vi "VI Main 1.2.vi"() -> ()   [LabVIEW 2014]
uses:
  <vilib>/Analysis/NI_AALPro.lvlib
panel:
  in  "Array":bool[](array[boolean])
  out "None linear Intervals":dbl[](array[numeric])
  out "Measuring! 2":bool
  in  "Residue Threshold":dbl=2.0 format="%.3g"
  in  "Gain":dbl=3.31
  in  "Offset":dbl=-0.032 step=0.01 format="%_3f"
  in  "K1":dbl=-2.995 format="%#_13g"
  in  "K0":dbl=0.9054 format="%#_13g"
  in  "samples/channel":i32=10
  in  "Rate (Hz)":dbl=100.0
  in  "DAQ channels":tag="Dev2/ai23"
  in  "RH/T Sensor VSS (V)":dbl=2.0 format="%.3g"
  out "residue":dbl
  in  "COM:":bool
  in  "clear graph at start":bool=TRUE
  in  "clear graph":bool
  out "Elapsed Time":dbl=5.100291728973389 format="%<%H:%M:%S>t"
  out "Measuring!":bool
  out "Current Interval":i32=2
  out "Benchmark (s)":dbl=1.077 format="%.2g"
  out "Start time":timestamp=timestamp(3634319869.0891385 s since 1904-01-01)
  in  "STOP acq":bool
  in  "# of Intervals":i32=20 min=2 step=1
  in  "Interval (s)":dbl=3.0 min=1.0 step=1.0
  in  "Quick Acq":bool
  in  "Multi Acq":bool
  in  "Reset":bool
  in  "Single Acq":bool
  in  "stop":bool
  out "intercept":dbl=5.632151768673284e-07 format="%_4g"
  out "Waveform Chart":dbl(graph)
  out "Res. (ohm)":dbl=1498.8953969009954 format="%#.5g"
  out "XY Graph":cluster{dbl[], "Best Linear Fit":dbl[]}[](graph)=[{[0.0, 0.05050000175833702, 0.10100000351667404, 0.15150000154972076, 0.20200000703334808, 0.2524999976158142, 0.30300000309944153, 0.35350000858306885, 0.40400001406669617, 0.4544999897480011, 0.5049999952316284, 0.5554999709129333, 0.6060000061988831, 0.656499981880188, 0.7070000171661377, 0.7574999928474426, 0.8080000281333923, 0.8585000038146973, 0.9089999794960022, 0.9595000147819519, 1.0099999904632568, 1.0605000257492065, 1.1109999418258667, 1.1614999771118164, 1.2120000123977661, 1.2625000476837158, 1.312999963760376, 1.3634999990463257, 1.4140000343322754, 1.4644999504089355, 1.5149999856948853, 1.565500020980835, 1.6160000562667847, 1.6664999723434448, 1.7170000076293945, 1.7675000429153442, 1.8179999589920044, 1.868499994277954, 1.9190000295639038, 1.969499945640564, 2.0199999809265137, 2.070499897003174, 2.121000051498413, 2.1714999675750732, 2.2219998836517334, 2.2725000381469727, 2.322999954223633, 2.373500108718872, 2.4240000247955322, 2.4744999408721924, 2.5255000591278076, 2.5759999752044678, 2.626499891281128, 2.677000045776367, 2.7274999618530273, 2.7780001163482666, 2.8285000324249268, 2.878999948501587, 2.929500102996826, 2.9800000190734863, 3.0304999351501465, 3.0810000896453857, 3.131500005722046, 3.181999921798706, 3.2325000762939453, 3.2829999923706055, 3.3334999084472656, 3.384000062942505, 3.434499979019165, 3.484999895095825, 3.5355000495910645, 3.5859999656677246, 3.6364998817443848, 3.687000036239624, 3.737499952316284, 3.7880001068115234, 3.8385000228881836, 3.8889999389648438, 3.939500093460083, 3.990000009536743, 4.040500164031982, 4.091000080108643, 4.141499996185303, 4.191999912261963, 4.242499828338623, 4.293000221252441, 4.343500137329102, 4.394000053405762, 4.444499969482422, 4.494999885559082, 4.545499801635742, 4.5960001945495605, 4.646500110626221, 4.697000026702881, 4.747499942779541, 4.797999858856201, 4.848499774932861, 4.89900016784668, 4.94950008392334, 5.0], "Best Linear Fit"=[2.9321361694201187e-07, 3.4316144592594355e-05, 6.788442260585725e-05, 0.00010163152910536155, 0.0001353666593786329, 0.0001692490477580577, 0.00020289691747166216, 0.0002365230757277459, 0.0002702110796235502, 0.0003039317671209574, 0.0003375497763045132, 0.00037135041202418506, 0.00040501810144633055, 0.000438651826698333, 0.0004723611054942012, 0.0005059913382865489, 0.0005397166823968291, 0.0005734616424888372, 0.0006071235402487218, 0.0006408520275726914, 0.000674474285915494, 0.0007079437491483986, 0.0007418016903102398, 0.0007753406534902751, 0.0008092316566035151, 0.0008428616565652192, 0.0008766247192397714, 0.0009101884788833559, 0.0009441068395972252, 0.000977773917838931, 0.0010113242315128446, 0.00104525254573673, 0.0010786742204800248, 0.0011119291884824634, 0.0011458882363513112, 0.0011792887235060334, 0.0012128128437325358, 0.001246674102731049, 0.0012809749459847808, 0.0013138956855982542, 0.0013484194641932845, 0.0013821402098983526, 0.001415521022863686, 0.0014488088199868798, 0.0014823464443907142, 0.0015171199338510633, 0.0015507071511819959, 0.0015843959990888834, 0.0016174258198589087, 0.001652282546274364, 0.001685628667473793, 0.001718429964967072, 0.0017526380252093077, 0.0017857326893135905, 0.0018194534350186586, 0.001854273141361773, 0.0018880483694374561, 0.0019207267323508859, 0.0019549881108105183, 0.001989204902201891, 0.0020224947948008776, 0.002056337194517255, 0.0020900650415569544, 0.0021233297884464264, 0.0021574627608060837, 0.0021917179692536592, 0.0022237151861190796, 0.002258580643683672, 0.0022912463173270226, 0.0023252873215824366, 0.0023596647661179304, 0.0023923530243337154, 0.0024269770365208387, 0.0024603772908449173, 0.002494191052392125, 0.0025280059780925512, 0.0025607654824852943, 0.0025952423457056284, 0.0026286595966666937, 0.0026625576429069042, 0.002696041017770767, 0.002730145351961255, 0.0027635691221803427, 0.0027978394646197557, 0.00283193145878613, 0.0028640953823924065, 0.002898684237152338, 0.0029313690029084682, 0.002965638181194663, 0.0029995907098054886, 0.0030326275154948235, 0.0030669174157083035, 0.003100987756624818, 0.003135110717266798, 0.0031680287793278694, 0.0032008818816393614, 0.0032355813309550285, 0.003269442357122898, 0.0033022440038621426, 0.0033363213296979666]}, {[0.0, 0.05050000175833702, 0.10100000351667404, 0.15150000154972076, 0.20200000703334808, 0.2524999976158142, 0.30300000309944153, 0.35350000858306885, 0.40400001406669617, 0.4544999897480011, 0.5049999952316284, 0.5554999709129333, 0.6060000061988831, 0.656499981880188, 0.7070000171661377, 0.7574999928474426, 0.8080000281333923, 0.8585000038146973, 0.9089999794960022, 0.9595000147819519, 1.0099999904632568, 1.0605000257492065, 1.1109999418258667, 1.1614999771118164, 1.2120000123977661, 1.2625000476837158, 1.312999963760376, 1.3634999990463257, 1.4140000343322754, 1.4644999504089355, 1.5149999856948853, 1.565500020980835, 1.6160000562667847, 1.6664999723434448, 1.7170000076293945, 1.7675000429153442, 1.8179999589920044, 1.868499994277954, 1.9190000295639038, 1.969499945640564, 2.0199999809265137, 2.070499897003174, 2.121000051498413, 2.1714999675750732, 2.2219998836517334, 2.2725000381469727, 2.322999954223633, 2.373500108718872, 2.4240000247955322, 2.4744999408721924, 2.5255000591278076, 2.5759999752044678, 2.626499891281128, 2.677000045776367, 2.7274999618530273, 2.7780001163482666, 2.8285000324249268, 2.878999948501587, 2.929500102996826, 2.9800000190734863, 3.0304999351501465, 3.0810000896453857, 3.131500005722046, 3.181999921798706, 3.2325000762939453, 3.2829999923706055, 3.3334999084472656, 3.384000062942505, 3.434499979019165, 3.484999895095825, 3.5355000495910645, 3.5859999656677246, 3.6364998817443848, 3.687000036239624, 3.737499952316284, 3.7880001068115234, 3.8385000228881836, 3.8889999389648438, 3.939500093460083, 3.990000009536743, 4.040500164031982, 4.091000080108643, 4.141499996185303, 4.191999912261963, 4.242499828338623, 4.293000221252441, 4.343500137329102, 4.394000053405762, 4.444499969482422, 4.494999885559082, 4.545499801635742, 4.5960001945495605, 4.646500110626221, 4.697000026702881, 4.747499942779541, 4.797999858856201, 4.848499774932861, 4.89900016784668, 4.94950008392334, 5.0], "Best Linear Fit"=[5.632151768673284e-07, 3.425469348999516e-05, 6.794617180312299e-05, 0.00010163764763089373, 0.00013532912842937865, 0.0001690205992864352, 0.00020271208008492013, 0.00023640356088340506, 0.00027009504168188996, 0.0003037865025975182, 0.0003374779833960031, 0.00037116944431163135, 0.0004048609449929729, 0.00043855240590860115, 0.0004722439065899428, 0.000505935367505571, 0.0005396268681869126, 0.0005733183291025409, 0.0006070097900181691, 0.0006407012906995107, 0.0006743927516151388, 0.0007080842522964805, 0.0007417756734463953, 0.0007754671741277369, 0.0008091586748090786, 0.0008428501754904202, 0.000876541596640335, 0.0009102330973216766, 0.0009439245980030183, 0.000977616019152933, 0.0010113075198342747, 0.0010449990205156163, 0.001078690521196958, 0.0011123819423468728, 0.0011460734430282144, 0.001179764943709556, 0.0012134563648594707, 0.0012471478655408123, 0.001280839366222154, 0.0013145307873720688, 0.0013482222880534104, 0.0013819137092033252, 0.0014156052894160936, 0.0014492967105660085, 0.0014829881317159233, 0.0015166797119286917, 0.0015503711330786066, 0.001584062713291375, 0.0016177541344412898, 0.0016514455555912046, 0.0016854706906080038, 0.0017191621117579187, 0.0017528535329078335, 0.001786545113120602, 0.0018202365342705167, 0.0018539281144832852, 0.0018876195356332, 0.0019213109567831148, 0.001955002536995883, 0.001988693958145798, 0.0020223853792957127, 0.0020560769595084813, 0.002089768380658396, 0.002123459801808311, 0.002157151382021079, 0.0021908428031709943, 0.002224534224320909, 0.0022582258045336775, 0.002291917225683592, 0.002325608646833507, 0.0023593002270462754, 0.00239299164819619, 0.002426683069346105, 0.0024603746495588733, 0.0024940660707087883, 0.0025277576509215565, 0.0025614490720714716, 0.002595140493221386, 0.002628832073434155, 0.0026625234945840694, 0.002696215074796838, 0.0027299064959467527, 0.0027635979170966677, 0.0027972893382465823, 0.0028309807593964974, 0.002864672498672119, 0.0028983639198220342, 0.002932055340971949, 0.002965746762121864, 0.0029994381832717785, 0.0030331296044216935, 0.0030668213436973154, 0.0031005127648472304, 0.003134204185997145, 0.0031678956071470596, 0.0032015870282969747, 0.0032352784494468893, 0.0032689701887225115, 0.003302661609872426, 0.003336353031022341]}]
  in  "Sense range":i32(slide)
  in  "Stop (V)":dbl=5.0 format="%.4f"
  in  "Source compliance (A)":dbl=0.01 format="%.4f"
  in  "Direction":i32(slide)
  in  "Ranging":i32(slide)
  in  "Start (V)":dbl step=1.0 format="%.4p"
  in  "# of points to acquire":i32=50 min=1 max=2500 step=1
  in  "Speed":i32(slide)=2
  out "status":i32 format="%.0x"
  in  "resource GPIB":string="GPIB0::24::INSTR"
  in  "resource RS232":string="ASRL4::INSTR"
  out "Qrun":bool
  out "Mrun":bool
  out "Srun":bool
  # ">"
  # "RH%/T Sensor"
  # "Ethanol Sensor"
  # "by L.Andrzejewski\nlandrzej@uottawa.ca"
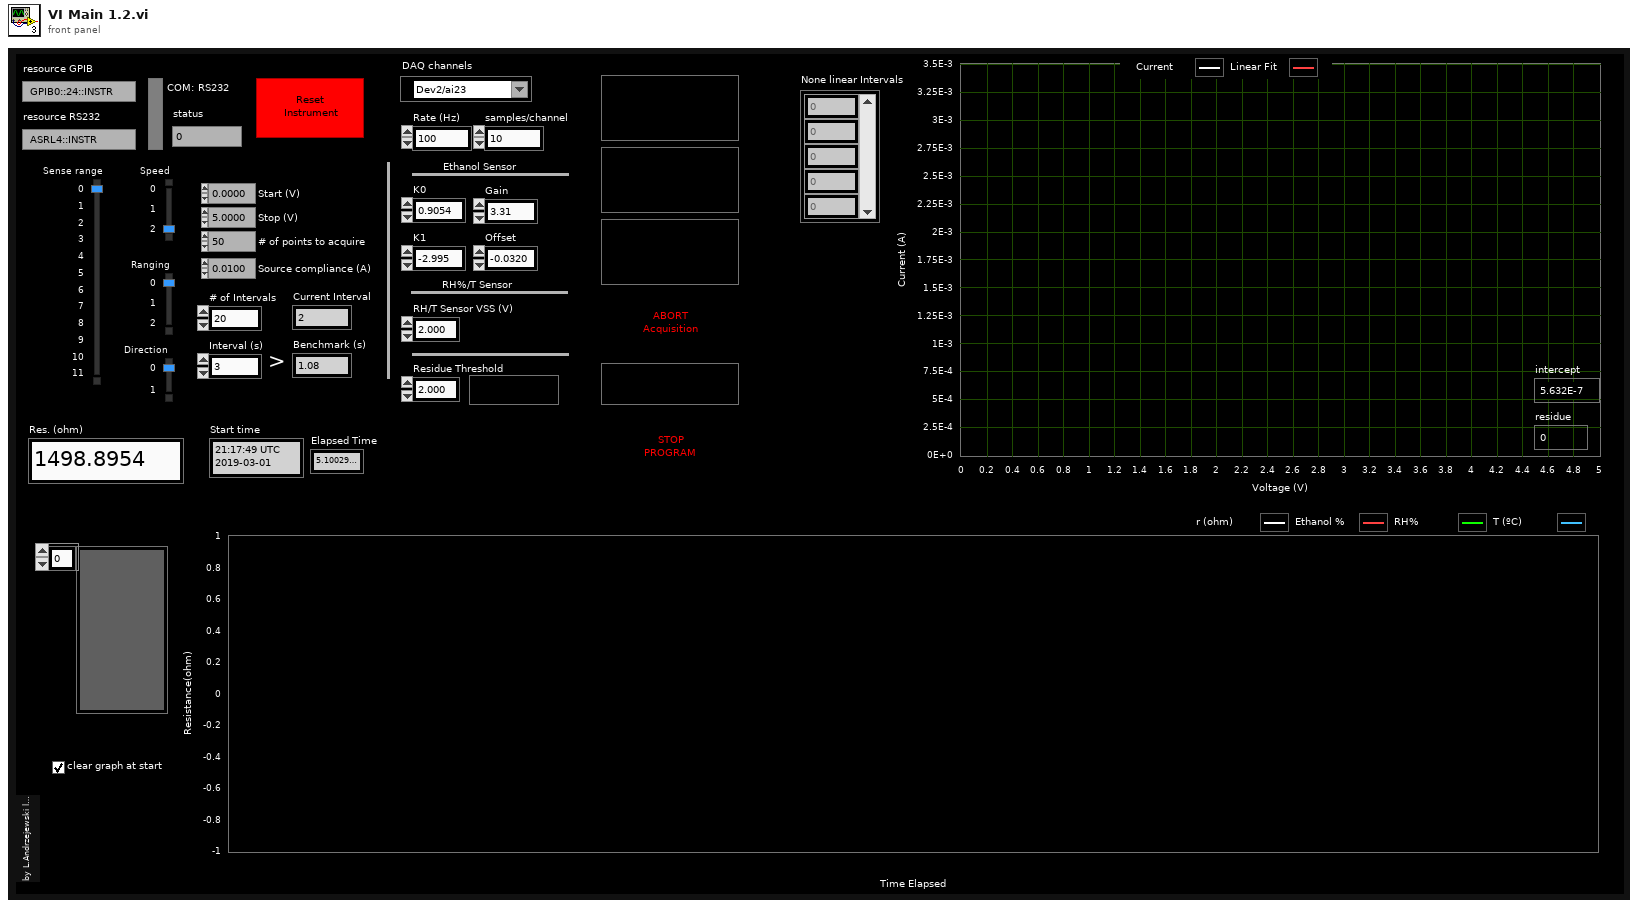
[diagram p1: front panel]
types:
  T1 = enum8{"Enabled", "Disabled", "Disabled and Grayed Out"}
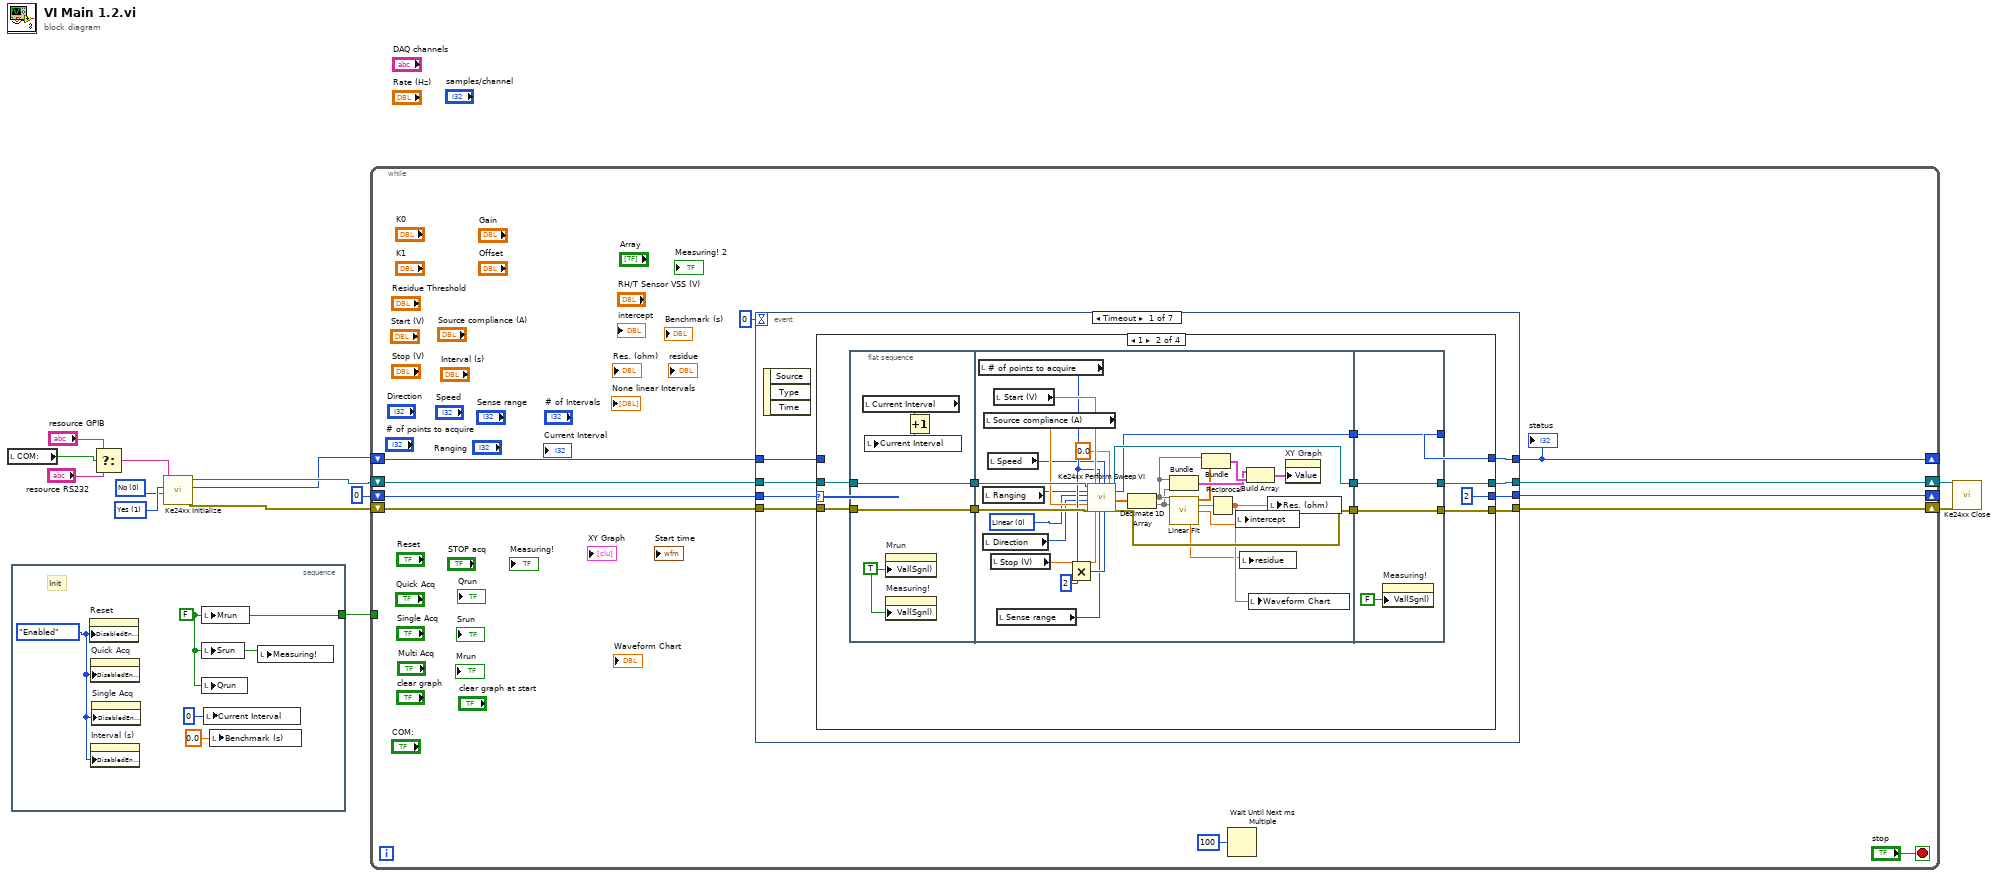
[diagram p0: block diagram]
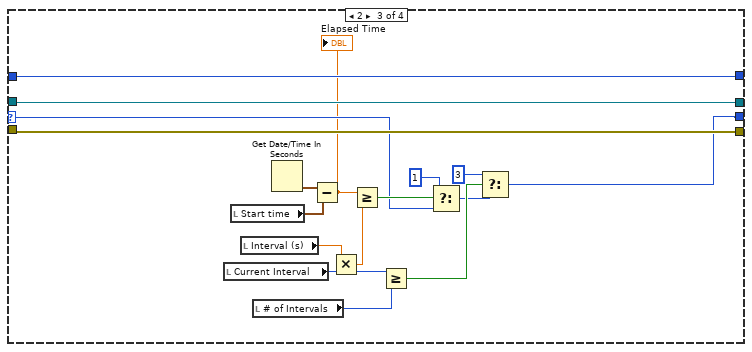
[diagram p3: hidden frame]
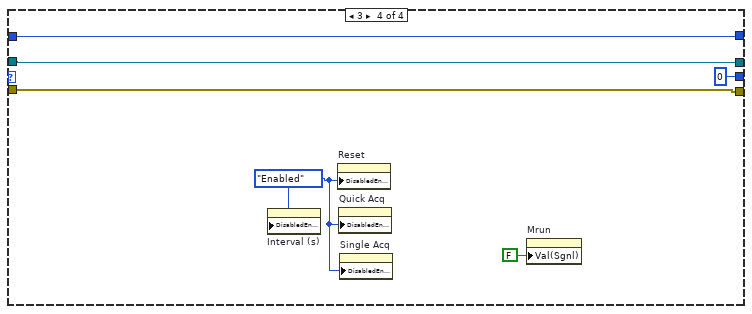
[diagram p4: hidden frame]
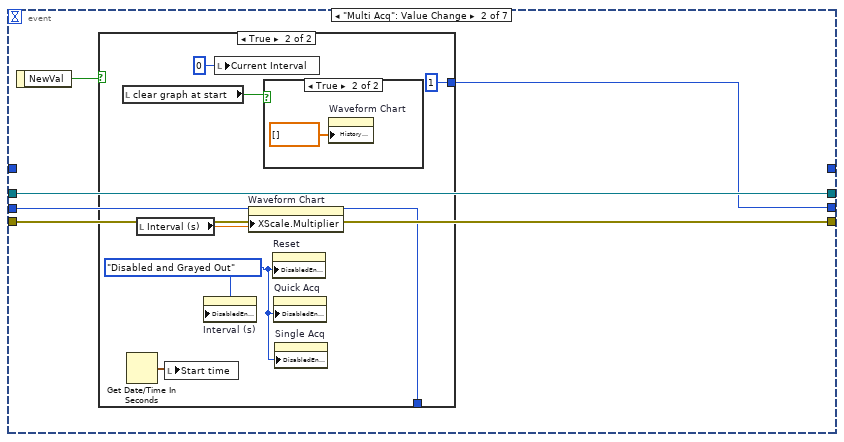
[diagram p5: hidden frame]
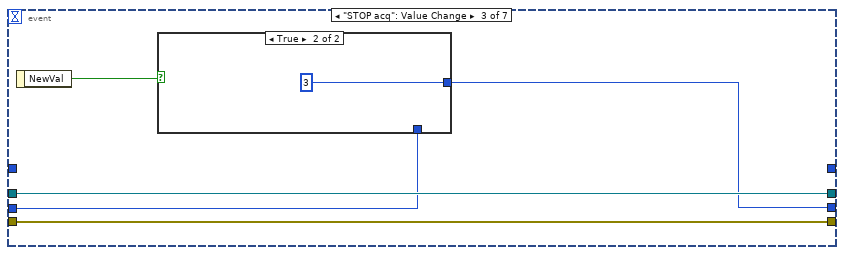
[diagram p8: hidden frame]
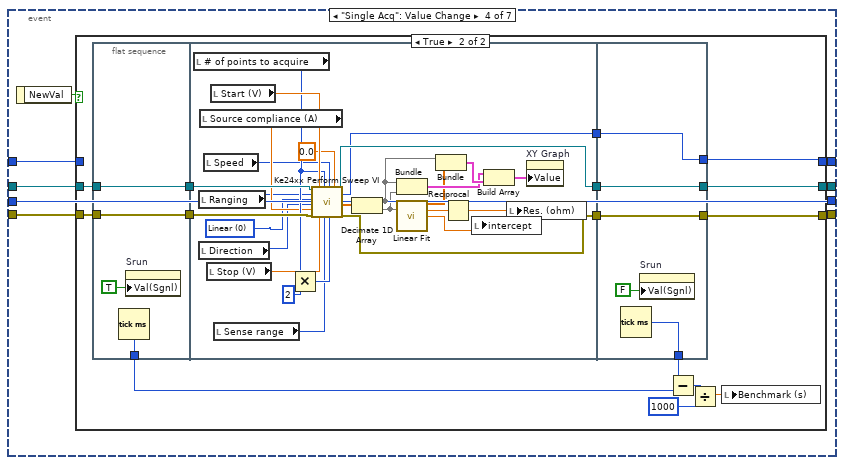
[diagram p10: hidden frame]
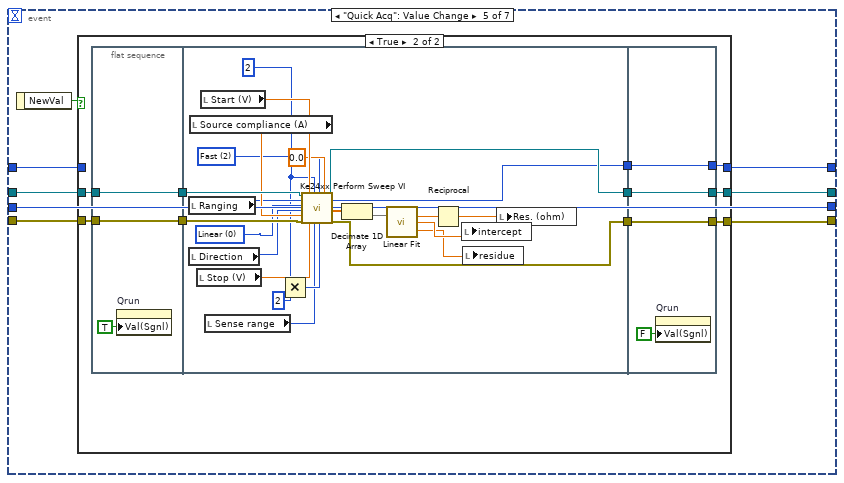
[diagram p12: hidden frame]
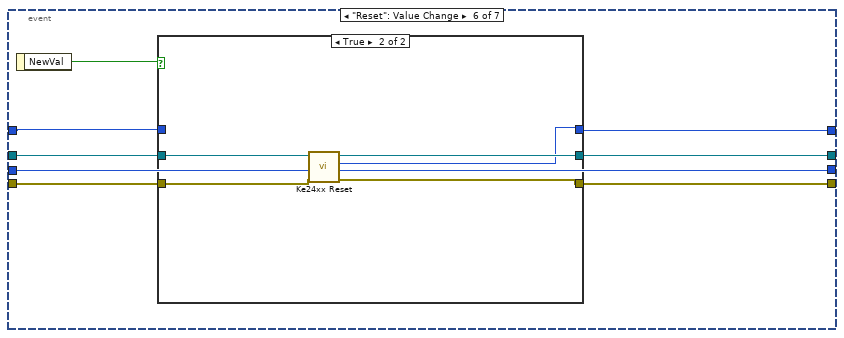
[diagram p14: hidden frame]
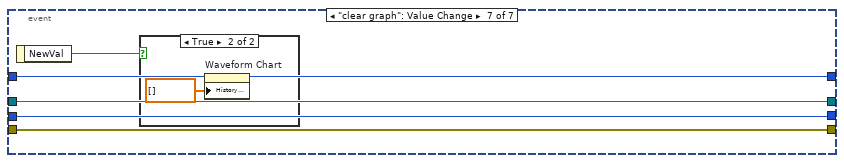
[diagram p16: hidden frame]
diagram:
  w13 = u16 1 items=["Yes"=1, "No"=0] ("id query")
  w5 = u16 0 items=["Yes"=1, "No"=0] ("reset device")
  n1 = local read "COM:"() -> (w4:bool)
  n2 = stacked-sequence {
    tunnel: [w15] -> w7
    frame #0 {
      w14 = T1."Enabled" ("Disabled")
      w15 = FALSE ("Mrun")
      # "Init"
      n3 = property on="Reset" class="Bool"("DisabledEnum"=w14) -> ()  [unwired: 2 in, 2 out]
      n4 = property on="Quick Acq" class="Bool"("DisabledEnum"=w14) -> ()  [unwired: 2 in, 2 out]
      n5 = property on="Interval (s)" class="DigNum (strict)"("DisabledEnum"=w14) -> ()  [unwired: 2 in, 2 out]
      n6 = property on="Single Acq" class="Bool"("DisabledEnum"=w14) -> ()  [unwired: 2 in, 2 out]
      n7 = local write "Mrun"(w15) -> ()
      n8 = local write "Srun"(w15) -> ()
      n9 = local write "Qrun"(w15) -> ()
      n10 = local write "Current Interval"(0 ("Current Interval")) -> ()
      n11 = local write "Benchmark (s)"(0.0 ("Benchmark (s)")) -> ()
      n12 = local write "Measuring!"(w15) -> ()
    }
  }
  n13 = Select(t="resource GPIB", s=w4, f="resource RS232") -> (s? t:f=w1:string)
  n14 = call <instrlib>:"Ke24xx Initialize.vi"("reset device"=w5, "id query"=w13, "resource name"=w1) -> ("error out"=w8:errorcluster, "status"=w9:i32, "instrument handle out"=w10:refnum<visa-resource-name>)  [unwired: 6 in]
  n15 = while {
    shift-right: [w23] -> w12
    shift-left: w10 -> [w25]
    shift-right: [w22] -> w11
    shift-left: w8 -> [w24]
    shift-right: [w20] -> _
    shift-left: w9 -> [w21]
    tunnel: w7 -> [_]
    shift-right: [w18] -> _
    shift-left: 0 -> [w19]
    stop <- "stop" stop-if-true
    n16 = event shown="[0] Timeout" {
      selector: _ -> [_ _ _ _ _ _ _]
      dyn-events: _ -> [_ _ _ _ _ _ _]
      timeout: 0 -> [_ _ _ _ _ _ _]
      tunnel: [w32 w115 w128 w135 w197 w249 w264] -> w23
      tunnel: w25 -> [w35 w115 w128 w138 w200 w250 w264]
      tunnel: [w31 w114 w127 w136 w198 w248 w262] -> w22
      tunnel: w24 -> [w34 w114 w127 w137 w199 w247 w262]
      tunnel: w21 -> [w33 _ _ w134 w196 w252 w265]
      tunnel: [w29 _ _ w133 w195 w251 w265] -> w20
      tunnel: w19 -> [w36 w112 w125 w132 w194 w246 w263]
      tunnel: [w30 w113 w126 w132 w194 w246 w263] -> w18
      event Timeout {
        n17 = event-data() -> ()  [unwired: 1 in, 3 out]
        n18 = case shown="1" w36 {
          selector: w36 -> [w37 _ w94 _]
          tunnel: w35 -> [w39 w49 w103 w109]
          tunnel: w34 -> [w38 w48 w104 w107]
          tunnel: w33 -> [w40 _ w105 w110]
          tunnel: [w39 w47 w103 w109] -> w32
          tunnel: [w38 w46 w104 w107] -> w31
          tunnel: [w37 2 w91 0 ("t")] -> w30
          tunnel: [w40 w44 w105 w110] -> w29
          frame 0, Default {
          }
          frame 1 {
            n19 = flat-sequence {
              tunnel: w48 -> [w55]
              tunnel: w49 -> [w56]
              tunnel: [w56] -> w51
              tunnel: [w55] -> w50
              tunnel: w51 -> [w77]
              tunnel: w50 -> [w76]
              tunnel: [w75] -> w43
              tunnel: [w74] -> w42
              tunnel: [w59] -> w41
              tunnel: [w86] -> w44
              tunnel: [w87] -> w47
              tunnel: [w88] -> w46
              tunnel: w43 -> [w88]
              tunnel: w42 -> [w87]
              tunnel: w41 -> [w86]
              frame #0 {
                w52 = TRUE ("Value (Signaling)")
                n20 = local read "Current Interval"() -> (w53:i32)
                n21 = property on="Mrun" class="Bool (strict)"("Val(Sgnl)"=w52) -> ()  [unwired: 2 in, 2 out]
                n22 = property on="Measuring!" class="Bool (strict)"("Val(Sgnl)"=w52) -> ()  [unwired: 2 in, 2 out]
                n23 = Increment(x=w53) -> (x+1=w54:i32)
                n24 = local write "Current Interval"(w54) -> ()
              }
              frame #1 {
                w61 = 0 items=["Linear", "Logarithmic"] ("spacing")
                n25 = local read "# of points to acquire"() -> (w68:i32)
                n26 = local read "Ranging"() -> (w63:i32)
                n27 = local read "Direction"() -> (w62:i32)
                n28 = local read "Source compliance (A)"() -> (w65:dbl)
                n29 = local read "Speed"() -> (w64:i32)
                n30 = local read "Stop (V)"() -> (w70:dbl)
                n31 = local read "Start (V)"() -> (w71:dbl)
                n32 = local read "Sense range"() -> (w66:i32)
                n33 = Multiply(x=w68, y=2) -> (x*y=w67:i32)
                n34 = call <instrlib>:"Ke24xx Perform Sweep VI.vi"("instrument handle"=w77, "ranging"=w63, "spacing"=w61, "direction"=w62, "source compliance"=w65, "error in (no error)"=w76, "start"=w71, "stop"=w70, "number of points"=w68, "sense range"=w66, "speed"=w64, "size of reading"=w67, "source protection"=0.0) -> ("instrument handle out"=w74:refnum<visa-resource-name>, "status"=w59:i32, "out"=w78:dbl[], "error out"=w75:errorcluster)  [unwired: 3 in]
                n35 = Decimate 1D Array(w78) -> (w82:dbl[], w79:dbl[])
                n36 = Bundle(w82, w79) -> (w83:cluster{dbl[], dbl[]})  [unwired: 1 in]
                n37 = call <vilib>:"Linear Fit.vi"("Y"=w79, "X"=w82) -> ("Best Linear Fit"=w81:dbl[], "slope"=w80:dbl, "intercept"=w73:dbl, "residue"=w57:dbl)  [unwired: 9 in, 1 out]
                n38 = Bundle(w82, "Best Linear Fit"=w81) -> (w84:cluster{dbl[], "Best Linear Fit":dbl[]})  [unwired: 1 in]
                n39 = Reciprocal(x=w80) -> (1/x=w58:dbl)
                n40 = local write "intercept"(w73) -> ()
                n41 = local write "residue"(w57) -> ()
                n42 = Build Array(w83, w84) -> (w72:cluster{dbl[], "Best Linear Fit":dbl[]}[])
                n43 = local write "Waveform Chart"(w58) -> ()
                n44 = local write "Res. (ohm)"(w58) -> ()
                n45 = property on="XY Graph" class="XYGraph (strict)"("Value"=w72) -> ()  [unwired: 2 in, 2 out]
              }
              frame #2 {
                n46 = property on="Measuring!" class="Bool (strict)"("Val(Sgnl)"=FALSE ("Value (Signaling)")) -> ()  [unwired: 2 in, 2 out]
              }
            }
          }
          frame 2 {
            n47 = local read "Current Interval"() -> (w97:i32)
            n48 = local read "Start time"() -> (w101:timestamp)
            n49 = local read "Interval (s)"() -> (w100:dbl)
            n50 = local read "# of Intervals"() -> (w96:i32)
            n51 = Get Date/Time In Seconds() -> (seconds since 1Jan1904=w102:timestamp)
            n52 = Subtract(x=w102, y=w101) -> (x-y=w89:dbl)
            "Elapsed Time" <- w89
            n53 = Multiply(x=w100, y=w97) -> (x*y=w99:dbl)
            n54 = Greater Or Equal?(x=w89, y=w99) -> (x >= y?=w98:bool)
            n55 = Greater Or Equal?(x=w97, y=w96) -> (x >= y?=w93:bool)
            n56 = Select(t=1, s=w98, f=w94) -> (s? t:f=w92:i32)
            n57 = Select(t=3, s=w93, f=w92) -> (s? t:f=w91:i32)
          }
          frame 3 {
            w106 = T1."Enabled" ("Disabled")
            n58 = property on="Interval (s)" class="DigNum (strict)"("DisabledEnum"=w106) -> ()  [unwired: 2 in, 2 out]
            n59 = property on="Reset" class="Bool"("DisabledEnum"=w106) -> ()  [unwired: 2 in, 2 out]
            n60 = property on="Quick Acq" class="Bool"("DisabledEnum"=w106) -> ()  [unwired: 2 in, 2 out]
            n61 = property on="Single Acq" class="Bool"("DisabledEnum"=w106) -> ()  [unwired: 2 in, 2 out]
            n62 = property on="Mrun" class="Bool (strict)"("Val(Sgnl)"=FALSE ("Value (Signaling)")) -> ()  [unwired: 2 in, 2 out]
          }
        }
      }
      event "Multi Acq": Value Change {
        n63 = event-data() -> ("NewVal"=w116:bool)  [unwired: 1 in]
        n64 = case shown="True" w116 {
          tunnel: [w117 1] -> w113
          tunnel: w112 -> [w117 _]
          frame False {
          }
          frame True {
            w119 = T1."Disabled and Grayed Out" ("Disabled")
            n65 = local read "clear graph at start"() -> (w118:bool)
            n66 = Get Date/Time In Seconds() -> (seconds since 1Jan1904=w121:timestamp)
            n67 = local read "Interval (s)"() -> (w120:dbl)
            n68 = local write "Start time"(w121) -> ()
            n69 = property on="Interval (s)" class="DigNum (strict)"("DisabledEnum"=w119) -> ()  [unwired: 2 in, 2 out]
            n70 = local write "Current Interval"(0 ("Current Interval")) -> ()
            n71 = property on="Waveform Chart" class="WFChart (strict)"("XScale.Multiplier"=w120) -> ()  [unwired: 2 in, 2 out]
            n72 = case shown="True" w118 {
              frame False {
              }
              frame True {
                n73 = property on="Waveform Chart" class="WFChart (strict)"("History Data"=dbl[] []) -> ()  [unwired: 2 in, 2 out]
              }
            }
            n74 = property on="Reset" class="Bool"("DisabledEnum"=w119) -> ()  [unwired: 2 in, 2 out]
            n75 = property on="Quick Acq" class="Bool"("DisabledEnum"=w119) -> ()  [unwired: 2 in, 2 out]
            n76 = property on="Single Acq" class="Bool"("DisabledEnum"=w119) -> ()  [unwired: 2 in, 2 out]
          }
        }
      }
      event "STOP acq": Value Change {
        n77 = event-data() -> ("NewVal"=w129:bool)  [unwired: 1 in]
        n78 = case shown="True" w129 {
          tunnel: [w130 3] -> w126
          tunnel: w125 -> [w130 _]
          frame False {
          }
          frame True {
          }
        }
      }
      event "Single Acq": Value Change {
        n79 = event-data() -> ("NewVal"=w139:bool)  [unwired: 1 in]
        n80 = case shown="True" w139 {
          tunnel: w138 -> [w142 w157]
          tunnel: w137 -> [w141 w156]
          tunnel: [w141 w155] -> w136
          tunnel: [w142 w154] -> w135
          tunnel: [w140 w149] -> w133
          tunnel: w134 -> [w140 _]
          frame False {
          }
          frame True {
            n81 = flat-sequence {
              tunnel: w156 -> [w160]
              tunnel: w157 -> [w161]
              tunnel: [w161] -> w151
              tunnel: [w160] -> w150
              tunnel: [w158] -> w146
              tunnel: [w179] -> w153
              tunnel: [w178] -> w152
              tunnel: w151 -> [w181]
              tunnel: w150 -> [w180]
              tunnel: [w162] -> w148
              tunnel: [w192] -> w154
              tunnel: [w193] -> w155
              tunnel: w153 -> [w193]
              tunnel: w152 -> [w192]
              tunnel: [w191] -> w149
              tunnel: w148 -> [w191]
              tunnel: [w189] -> w147
              frame #0 {
                n82 = Tick Count (ms)() -> (millisecond timer value=w158:u32)
                n83 = property on="Srun" class="Bool (strict)"("Val(Sgnl)"=TRUE ("Value (Signaling)")) -> ()  [unwired: 2 in, 2 out]
              }
              frame #1 {
                w164 = 0 items=["Linear", "Logarithmic"] ("spacing")
                n84 = local read "# of points to acquire"() -> (w171:i32)
                n85 = local read "Ranging"() -> (w166:i32)
                n86 = local read "Direction"() -> (w165:i32)
                n87 = local read "Source compliance (A)"() -> (w168:dbl)
                n88 = local read "Speed"() -> (w167:i32)
                n89 = local read "Stop (V)"() -> (w173:dbl)
                n90 = local read "Start (V)"() -> (w174:dbl)
                n91 = local read "Sense range"() -> (w169:i32)
                n92 = Multiply(x=w171, y=2) -> (x*y=w170:i32)
                n93 = call <instrlib>:"Ke24xx Perform Sweep VI.vi"("instrument handle"=w181, "ranging"=w166, "spacing"=w164, "direction"=w165, "source compliance"=w168, "error in (no error)"=w180, "start"=w174, "stop"=w173, "number of points"=w171, "sense range"=w169, "speed"=w167, "size of reading"=w170, "source protection"=0.0) -> ("instrument handle out"=w178:refnum<visa-resource-name>, "status"=w162:i32, "out"=w182:dbl[], "error out"=w179:errorcluster)  [unwired: 3 in]
                n94 = Decimate 1D Array(w182) -> (w186:dbl[], w183:dbl[])
                n95 = Bundle(w186, w183) -> (w187:cluster{dbl[], dbl[]})  [unwired: 1 in]
                n96 = call <vilib>:"Linear Fit.vi"("Y"=w183, "X"=w186) -> ("Best Linear Fit"=w185:dbl[], "slope"=w184:dbl, "intercept"=w177:dbl)  [unwired: 9 in, 2 out]
                n97 = Bundle(w186, "Best Linear Fit"=w185) -> (w188:cluster{dbl[], "Best Linear Fit":dbl[]})  [unwired: 1 in]
                n98 = Reciprocal(x=w184) -> (1/x=w176:dbl)
                n99 = local write "intercept"(w177) -> ()
                n100 = Build Array(w187, w188) -> (w175:cluster{dbl[], "Best Linear Fit":dbl[]}[])
                n101 = local write "Res. (ohm)"(w176) -> ()
                n102 = property on="XY Graph" class="XYGraph (strict)"("Value"=w175) -> ()  [unwired: 2 in, 2 out]
              }
              frame #2 {
                n103 = Tick Count (ms)() -> (millisecond timer value=w189:u32)
                n104 = property on="Srun" class="Bool (strict)"("Val(Sgnl)"=FALSE ("Value (Signaling)")) -> ()  [unwired: 2 in, 2 out]
              }
            }
            n105 = Subtract(x=w147, y=w146) -> (x-y=w145:u32)
            n106 = Divide(x=w145, y=u32 1000) -> (x/y=w143:dbl)
            n107 = local write "Benchmark (s)"(w143) -> ()
          }
        }
      }
      event "Quick Acq": Value Change {
        n108 = event-data() -> ("NewVal"=w201:bool)  [unwired: 1 in]
        n109 = case shown="True" w201 {
          tunnel: w200 -> [w204 w214]
          tunnel: w199 -> [w203 w213]
          tunnel: [w203 w212] -> w198
          tunnel: [w204 w211] -> w197
          tunnel: [w202 w206] -> w195
          tunnel: w196 -> [w202 _]
          frame False {
          }
          frame True {
            n110 = flat-sequence {
              tunnel: w213 -> [w216]
              tunnel: w214 -> [w217]
              tunnel: [w217] -> w210
              tunnel: [w216] -> w209
              tunnel: w210 -> [w237]
              tunnel: w209 -> [w236]
              tunnel: [w235] -> w208
              tunnel: [w234] -> w207
              tunnel: [w220] -> w205
              tunnel: [w244] -> w211
              tunnel: [w245] -> w212
              tunnel: w208 -> [w245]
              tunnel: w207 -> [w244]
              tunnel: [w242] -> w206
              tunnel: w205 -> [w242]
              frame #0 {
                n111 = property on="Qrun" class="Bool (strict)"("Val(Sgnl)"=TRUE ("Qrun")) -> ()  [unwired: 2 in, 2 out]
              }
              frame #1 {
                w221 = 2 items=["Slow", "Medium", "Fast"] ("speed")
                w222 = 2 ("x")
                w224 = 0 items=["Linear", "Logarithmic"] ("spacing")
                n112 = local read "Ranging"() -> (w226:i32)
                n113 = local read "Direction"() -> (w225:i32)
                n114 = local read "Source compliance (A)"() -> (w227:dbl)
                n115 = local read "Stop (V)"() -> (w231:dbl)
                n116 = local read "Start (V)"() -> (w232:dbl)
                n117 = local read "Sense range"() -> (w228:i32)
                n118 = Multiply(x=w222, y=2) -> (x*y=w229:i32)
                n119 = call <instrlib>:"Ke24xx Perform Sweep VI.vi"("instrument handle"=w237, "ranging"=w226, "spacing"=w224, "direction"=w225, "source compliance"=w227, "error in (no error)"=w236, "start"=w232, "stop"=w231, "number of points"=w222, "sense range"=w228, "speed"=w221, "size of reading"=w229, "source protection"=0.0) -> ("instrument handle out"=w234:refnum<visa-resource-name>, "status"=w220:i32, "out"=w238:dbl[], "error out"=w235:errorcluster)  [unwired: 3 in]
                n120 = Decimate 1D Array(w238) -> (w241:dbl[], w239:dbl[])
                n121 = call <vilib>:"Linear Fit.vi"("Y"=w239, "X"=w241) -> ("slope"=w240:dbl, "intercept"=w233:dbl, "residue"=w218:dbl)  [unwired: 9 in, 2 out]
                n122 = Reciprocal(x=w240) -> (1/x=w219:dbl)
                n123 = local write "intercept"(w233) -> ()
                n124 = local write "residue"(w218) -> ()
                n125 = local write "Res. (ohm)"(w219) -> ()
              }
              frame #2 {
                n126 = property on="Qrun" class="Bool (strict)"("Val(Sgnl)"=FALSE ("Qrun")) -> ()  [unwired: 2 in, 2 out]
              }
            }
          }
        }
      }
      event "Reset": Value Change {
        n127 = event-data() -> ("NewVal"=w253:bool)  [unwired: 1 in]
        n128 = case shown="True" w253 {
          tunnel: [w256 w257] -> w251
          tunnel: w252 -> [w256 _]
          tunnel: w250 -> [w255 w261]
          tunnel: [w255 w260] -> w249
          tunnel: [w254 w258] -> w248
          tunnel: w247 -> [w254 w259]
          frame False {
          }
          frame True {
            n129 = call <instrlib>:"Ke24xx Reset.vi"("error in (no error)"=w259, "instrument handle"=w261) -> ("error out"=w258:errorcluster, "status"=w257:i32, "instrument handle out"=w260:refnum<visa-resource-name>)  [unwired: 7 in]
          }
        }
      }
      event "clear graph": Value Change {
        n130 = event-data() -> ("NewVal"=w266:bool)  [unwired: 1 in]
        n131 = case shown="True" w266 {
          frame False {
          }
          frame True {
            n132 = property on="Waveform Chart" class="WFChart (strict)"("History Data"=dbl[] []) -> ()  [unwired: 2 in, 2 out]
          }
        }
      }
    }
    "status" <- w20
    n133 = Wait Until Next ms Multiple(millisecond multiple=u32 100) -> ()  [unwired: 1 out]
  }
  n134 = call <instrlib>:"Ke24xx Close.vi"("error in (no error)"=w11, "instrument handle"=w12) -> ()  [unwired: 8 in, 2 out]
